vi "Shutdown.vi"(8 "error in":errorcluster, 11 "nPAS in":refnum<class "nPAS.lvclass">) -> (0 "error out":errorcluster, 3 "nPAS out":refnum<class "nPAS.lvclass">)   [LabVIEW 2014, in "nPAS.lvclass"]
doc: "Shutoff the DC power which will control all outputs, close all references to DAQmx tasks and shutoff the laser AO."
uses:
  nPAS.lvclass
  Session/Raw FPGA/FPGA Session.lvclass
  nPAS.lvclass/nPAS.ctl
  Reusable/PAS/Main/PAS.lvclass
  <userlib>/_Session Fwk/Session - Root.lvclass
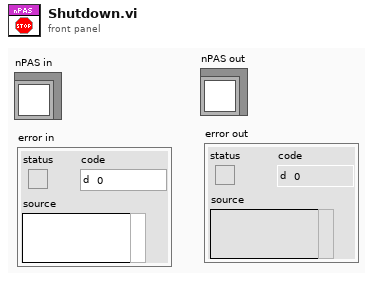
[diagram p1: front panel]
types:
  T1 = typedef "Session - Root.lvclass/Session Handle.ctl" = refnum<data-value>
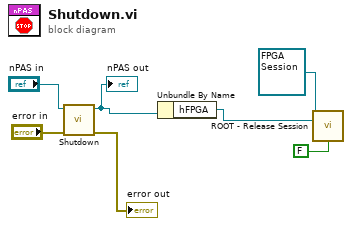
[diagram p0: block diagram]
diagram:
  n1 = call-parent "Shutdown.vi"("error in"="error in", "Instrument in"="nPAS in") -> ("error out"=→"error out":errorcluster, "Instrument out"=w4:refnum<class "nPAS.lvclass">)  [unwired: 8 in]
  "nPAS out" <- w4
  n2 = Unbundle By Name(w4) -> ("hFPGA"=w3:T1)
  n3 = call <userlib>:"ROOT - Release Session.vi"("OBJ - Session in"=refnum<class "FPGA Session.lvclass"> refnum ("FPGA Session"), "Session Handle in"=w3, "force destroy? (F)"=FALSE) -> ()  [unwired: 10 in, 3 out]
